vi "Read from File.vi"(8 "error in (no error)":errorcluster, 10 "INI Ref":T1, 11 "Control Assertion in":refnum<class "Control Assertion.lvclass">) -> (0 "error out":errorcluster, 2 "INI Ref out":T1, 3 "Control Assertion out":refnum<class "Control Assertion.lvclass">)   [LabVIEW 2020, in "MacroAssert.lvlib" / "Control Assertion.lvclass"]
uses:
  Control Assertion.lvclass
  C:/Users/User/Documents/LabVIEW Data/Projects/MacroAssert/source/Classes/Step/Step.lvclass
  <vilib>/Utility/config.llb/Config Data RefNum.ctl
  <vilib>/Utility/config.llb/Read Key (String).vi
  Assertion Step/Assertion Step.lvclass
  <vilib>/Utility/config.llb/NI_LVConfig.lvlib
  MacroAssert.lvlib
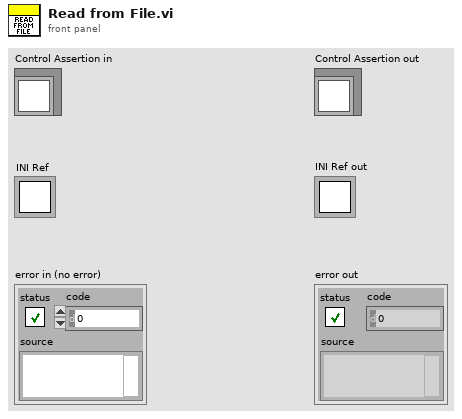
[diagram p1: front panel]
types:
  T1 = typedef "NI_LVConfig.lvlib/Config Data RefNum.ctl" = refnum<k1>
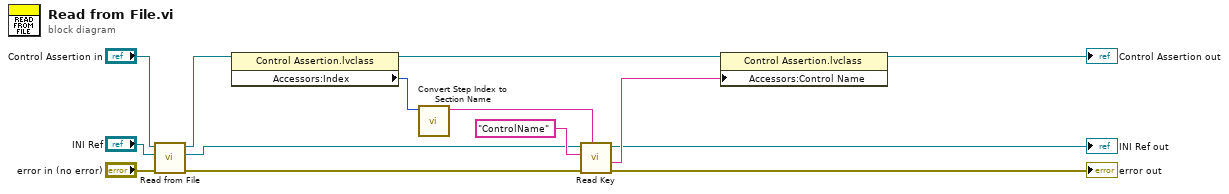
[diagram p0: block diagram]
diagram:
  n1 = call-parent "Read from File.vi"("error in (no error)"="error in (no error)", "INI Ref"="INI Ref", "Assertion Step in"="Control Assertion in") -> ("error out"=w6:errorcluster, "INI Ref out"=w5:T1, "Assertion Step out"=w4:refnum<class "Control Assertion.lvclass">)  [unwired: 6 in]
  n2 = property class="Control Assertion.lvclass"(reference=w4) -> (reference out=w9:refnum<class "Control Assertion.lvclass">, "Accessors:Index"=w8:i32)  [unwired: 1 in, 1 out]
  n3 = call "Convert Step Index to Section Name.vi"("Step Index"=w8) -> ("Section Name"=w7:string)  [unwired: 10 in]
  n4 = call-poly <vilib>:"Read Key.vi"("section"=w7, "error in (no error)"=w6, "key"="ControlName", "refnum"=w5) -> ("error out"=→"error out":errorcluster, "value"=w10:string, "refnum out"=→"INI Ref out":T1)  [unwired: 4 in, 1 out]
  n5 = property class="Control Assertion.lvclass"(reference=w9, "Accessors:Control Name"=w10) -> (reference out=→"Control Assertion out":refnum<class "Control Assertion.lvclass">)  [unwired: 1 in, 1 out]
